vi "Test pump WP calibration.vi"() -> ()   [LabVIEW 2013]
uses:
  <vilib>/Utility/file.llb/Write To Spreadsheet File (DBL).vi
panel:
  in  "Threshold":dbl
  out "WP calibration array":dbl[][](array[numeric])
  out "Photon #":dbl
  out "Max pump power":dbl
  in  "COM for WPs":u8=3
  in  "Manual?":bool
  in  "Blocking requirements":cluster{"Value":dbl, " Number":i32}[](array[cluster])
  out "error out":errorcluster
  in  "error in (no error)":errorcluster
  in  "Manual \nphoton #":i64=100
  in  "Target trigger\nrate (Hz)":dbl
  in  "Pump mode":enum16{"Constant power", "Constant time"}(ring)
  in  "Target trial \nlength (ms)":dbl=500.0 format="%.2p"
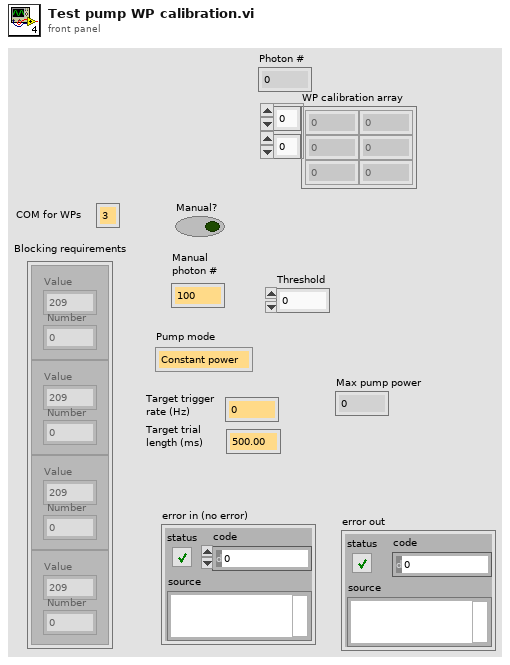
[diagram p1: front panel]
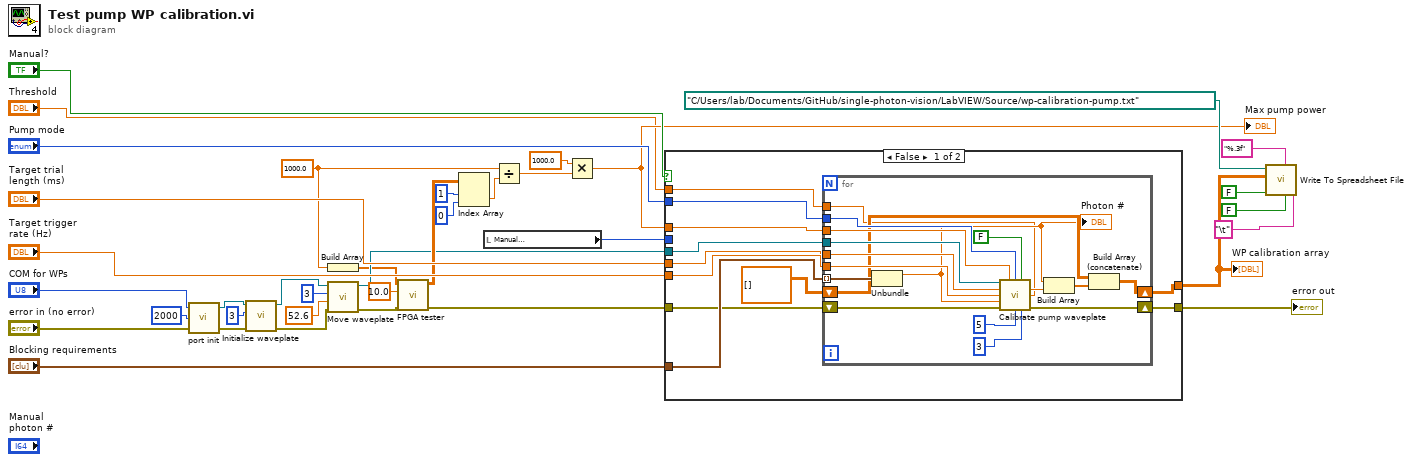
[diagram p0: block diagram]
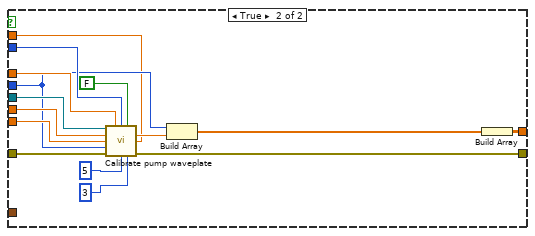
[diagram p2: hidden frame]
diagram:
  w5 = 1000.0 ("element")
  n1 = call "port init.vi"("error in"="error in (no error)", "Timeout (ms)"=u32 2000 ("Timeout (300 ms)"), "SerialPort"="COM for WPs") -> ("error out"=w16:errorcluster, "Visa Handle"=w15:refnum<visa-resource-name>)  [unwired: 1 in]
  n2 = call "Initialize waveplate.vi"("error in (no error)"=w16, "Axis in"=3, "VISA Handle in"=w15) -> ("error out"=w12:errorcluster, "VISA Refnum out"=w9:refnum<visa-resource-name>)  [unwired: 6 in, 1 out]
  n3 = Build Array(w5) -> (w6:dbl[])
  n4 = call "Move waveplate.vi"("error in (no error)"=w12, "Angle"=52.6, "Axis in"=3, "VISA Refnum in"=w9) -> ("error out"=w29:errorcluster, "VISA Refnum out"=w28:refnum<visa-resource-name>)  [unwired: 4 in, 2 out]
  n5 = call "FPGA tester.vi"("error in"=w29, "Repetitions"=10.0, "Levels"=w6) -> ("error out"=w34:errorcluster, "Results"=w32:dbl[][])  [unwired: 3 in]
  n6 = Index Array(array=w32, index (row)=1, index (col)=0 ("disabled index (col)")) -> (element=w8:dbl)
  n7 = local read "Manual \nphoton #"() -> (w25:i64)
  n8 = Divide(x=w5, y=w8) -> (x/y=w7:dbl)
  n9 = Multiply(x=1000.0, y=w7) -> (x*y=w3:dbl)
  "Max pump power" <- w3
  n10 = case shown="False" "Manual?" {
    tunnel: "Target trigger\nrate (Hz)" -> [w48 w80]
    tunnel: "Target trial \nlength (ms)" -> [w47 w79]
    tunnel: "Pump mode" -> [w46 w78]
    tunnel: "Blocking requirements" -> [w45 _]
    tunnel: [w44 w77] -> w19
    tunnel: w34 -> [w43 w76]
    tunnel: w3 -> [w42 w75]
    tunnel: w28 -> [w41 w74]
    tunnel: w25 -> [_ w73]
    tunnel: [w40 w67] -> w2
    tunnel: "Threshold" -> [w39 w66]
    frame False {
      n11 = for {
        tunnel: w48 -> [w65]
        tunnel: w47 -> [w64]
        tunnel: w46 -> [w63]
        tunnel: w45 -> [w62] mode=indexing
        shift-right: [w60] -> w44
        shift-left: w43 -> [w61]
        tunnel: w41 -> [w59]
        tunnel: w42 -> [w55]
        shift-right: [w52] -> w40
        shift-left: dbl[][] [] -> [w51]
        tunnel: w39 -> [w49]
        n12 = Unbundle(w62) -> ("Value"=w50:dbl)  [unwired: 1 out]
        "Photon #" <- w50
        n13 = call "Calibrate pump waveplate.vi"("VISA Refnum in"=w59, "Trigger rate \nat maximum"=w55, "Mode"=w63, "Trigger rate warnings?"=FALSE, "Target trial \nlength (ms)"=w64, "Target trigger rate"=w65, "Threshold"=w49, "Photon #"=w50, "error in (no error)"=w61, "N"=5, "Axis in"=3) -> ("WP position"=w54:dbl, "error out"=w60:errorcluster)  [unwired: 1 in, 2 out]
        n14 = Build Array(w50, w54) -> (w53:dbl[])
        n15 = Build Array (concatenate)(w51, w53) -> (w52:dbl[][])
      }
    }
    frame True {
      n16 = call "Calibrate pump waveplate.vi"("VISA Refnum in"=w74, "Trigger rate \nat maximum"=w75, "Mode"=w78, "Trigger rate warnings?"=FALSE, "Target trial \nlength (ms)"=w79, "Target trigger rate"=w80, "Threshold"=w66, "Photon #"=w73, "error in (no error)"=w76, "N"=5, "Axis in"=3) -> ("WP position"=w69:dbl, "error out"=w77:errorcluster)  [unwired: 1 in, 2 out]
      n17 = Build Array(w73, w69) -> (w68:dbl[])
      n18 = Build Array(w68) -> (w67:dbl[][])
    }
  }
  "error out" <- w19
  "WP calibration array" <- w2
  n19 = call-poly <vilib>:"Write To Spreadsheet File.vi"("delimiter (\\t)"="\t" ("delimiter (\\t)"), "transpose? (no:F)"=FALSE, "format (%.3f)"="%.3f", "append to file? (new file:F)"=FALSE, "2D data"=w2, "file path (dialog if empty)"=path "C:/Users/lab/Documents/GitHub/single-photon-vision/LabVIEW/Source/wp-calibration-pump.txt") -> ()  [unwired: 2 in, 1 out]
